vi "Transmission.vi"(9 "Buttons":bool[](array[boolean]), 10 "Axes":dbl[](array[numeric]), 11 "SolenoidDevRef":T1={"DevStatus"={"status"=FALSE, "code"=0, "source"=""}, "Pneumatics Control Module"=0, "Forward Solenoid Channel"=enum."Invalid", "Reverse Solenoid Channel"=enum."Invalid"}) -> ()   [LabVIEW 2014]
uses:
  <vilib>/Rock Robotics/WPI/Solenoid/WPI_SolenoidDevRef.ctl
  <vilib>/Rock Robotics/WPI/Solenoid/WPI_SolenoidChannel.ctl
  <vilib>/Rock Robotics/WPI/Solenoid/WPI_SolenoidValue.ctl
  <vilib>/Rock Robotics/WPI/Solenoid/WPI_SolenoidSetEnum.vi
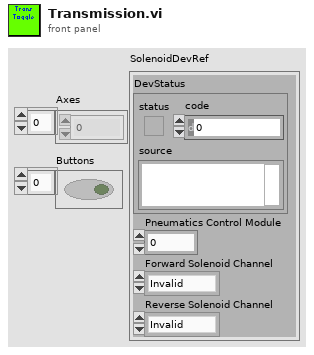
[diagram p1: front panel]
types:
  T1 = typedef "WPI_SolenoidDevRef.ctl" = cluster{"DevStatus":errorcluster, "Pneumatics Control Module":u8, "Forward Solenoid Channel":T2, "Reverse Solenoid Channel":T2}
  T2 = typedef "WPI_SolenoidChannel.ctl" = enum8{"Solenoid 0", "Solenoid 1", "Solenoid 2", "Solenoid 3", "Solenoid 4", "Solenoid 5", "Solenoid 6", "Solenoid 7", "Invalid"}
  T3 = typedef "WPI_SolenoidValue.ctl" = enum16{"Off", "On", "Forward", "Reverse"}
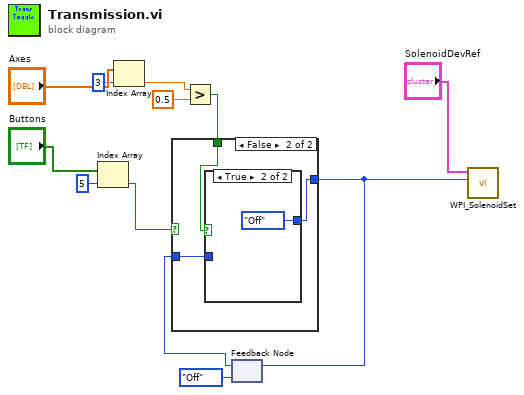
[diagram p0: block diagram]
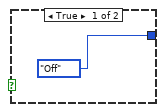
[diagram p2: hidden frame]
diagram:
  n1 = Index Array(array="Buttons", index=5) -> (element=w9:bool)
  n2 = Index Array(array="Axes", index=3) -> (element=w6:dbl)
  n3 = Greater?(x=w6, y=0.5) -> (0:w4:bool)
  n4 = feedback #1(WPI_SolenoidValue."Off" ("Value")) -> (w2:T3)
  n5 = case shown="False" w9 {
    tunnel: w4 -> [_ w16]
    tunnel: [WPI_SolenoidValue."Off" ("Value") w14] -> w3
    tunnel: w2 -> [_ w15]
    frame True {
    }
    frame False {
      n6 = case shown="True" w16 {
        tunnel: w15 -> [w17 _]
        tunnel: [w17 WPI_SolenoidValue."Off" ("Value")] -> w14
        frame False {
        }
        frame True {
        }
      }
    }
  }
  n7 = feedback-in #1(w3) -> ()
  n8 = call-poly <vilib>:"WPI_SolenoidSet.vi"("Value"=w3, "SolenoidDevRef"="SolenoidDevRef") -> ()  [unwired: 8 in, 2 out]
